vi "DSF.Engine.Plugin.Tx.Inline.Wait.vi"(8 "error in (no error)":errorcluster, 11 "Plugin in":refnum<class "DSF.Engine.Plugin.lvclass">) -> (0 "error out":errorcluster, 3 "Plugin out":refnum<class "DSF.Engine.Plugin.lvclass">)   [LabVIEW 2017, in "DSF.Engine.lvlib" / "DSF.Engine.Plugin.lvclass"]
uses:
  DSF.Engine.Plugin.lvclass
  DSF.Engine.Plugin.lvclass/DSF.Engine.Plugin.ctl
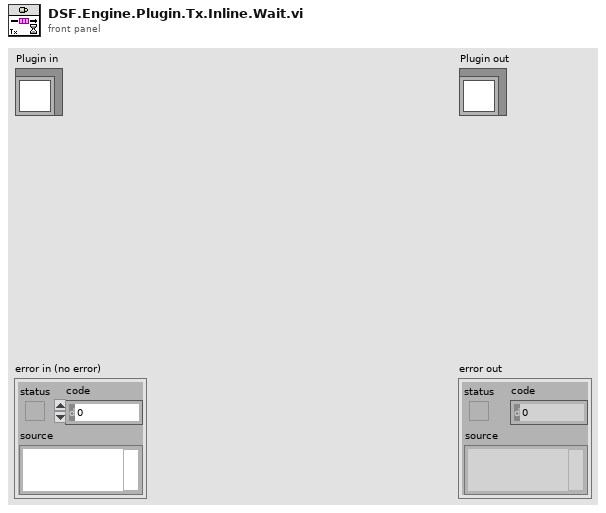
[diagram p1: front panel]
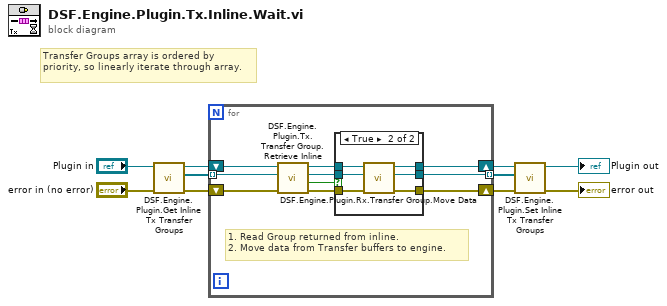
[diagram p0: block diagram]
diagram:
  # "Transfer Groups array is ordered by priority, so linearly iterate through array."
  n1 = call "DSF.Engine.Plugin.Get Inline Tx Transfer Groups.vi"("Plugin in"="Plugin in") -> ("Inline Tx Transfer Groups"=w8:refnum<class "DSF.Engine.Transfer Group.lvclass">[], "Plugin out"=w7:refnum<class "DSF.Engine.Plugin.lvclass">)  [unwired: 9 in]
  n2 = for {
    tunnel: w8 -> [w12] mode=indexing
    shift-right: [w11] -> w6
    shift-left: w7 -> [w14]
    shift-right: [w9] -> w2
    shift-left: "error in (no error)" -> [w13]
    tunnel: [w10] -> w5 mode=indexing
    # "1. Read Group returned from inline.\n2. Move data from Transfer buffers to engine."
    n3 = call "DSF.Engine.Plugin.Tx.Transfer Group.Retrieve Inline.vi"("error in (no error)"=w13, "Transfer Group in"=w12, "Plugin in"=w14) -> ("error out"=w15:errorcluster, "move data?"=w16:bool, "Transfer Group out"=w17:refnum<class "DSF.Engine.Transfer Group.lvclass">, "Plugin out"=w18:refnum<class "DSF.Engine.Plugin.lvclass">)  [unwired: 5 in]
    n4 = case shown="True" w16 {
      tunnel: w18 -> [w20 w27]
      tunnel: w17 -> [w21 w26]
      tunnel: [w20 w25] -> w11
      tunnel: [w21 w24] -> w10
      tunnel: [w19 w23] -> w9
      tunnel: w15 -> [w19 w22]
      frame False {
      }
      frame True {
        n5 = call "DSF.Engine.Plugin.Rx.Transfer Group.Move Data.vi"("error in (no error)"=w22, "Transfer Group in"=w26, "Plugin in"=w27) -> ("error out"=w23:errorcluster, "Transfer Group out"=w24:refnum<class "DSF.Engine.Transfer Group.lvclass">, "Plugin out"=w25:refnum<class "DSF.Engine.Plugin.lvclass">)  [unwired: 6 in]
      }
    }
  }
  "error out" <- w2
  n6 = call "DSF.Engine.Plugin.Set Inline Tx Transfer Groups.vi"("Inline Tx Transfer Groups"=w5, "Plugin in"=w6) -> ("Plugin out"=→"Plugin out":refnum<class "DSF.Engine.Plugin.lvclass">)  [unwired: 9 in]
